vi "calibrationSpectrometer_acceptCommand_Enable.vi"(8 "error in (no error)":errorcluster, 11 "command_Enable_Ctl":T1) -> (0 "error out":errorcluster, 2 "function return":i32, 3 "command_Enable_Ctl out":T1)   [LabVIEW 2016, in "SALLV_calibrationSpectrometer.lvlib"]
doc: "int calibrationSpectrometer_shm_acceptCommand_EnableLV(calibrationSpectrometer_command_EnableLV *command_Enable_Ctl );"
uses:
  SALLV_calibrationSpectrometer.lvlib
  DataTypes/command_Enable.ctl
  SALLV_calibrationSpectrometer.so
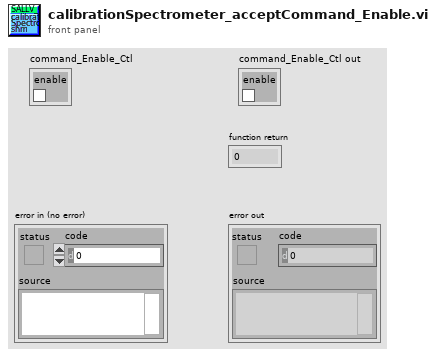
[diagram p1: front panel]
types:
  T1 = typedef "SALLV_calibrationSpectrometer.lvlib/command_Enable.ctl" = cluster{"enable":bool}
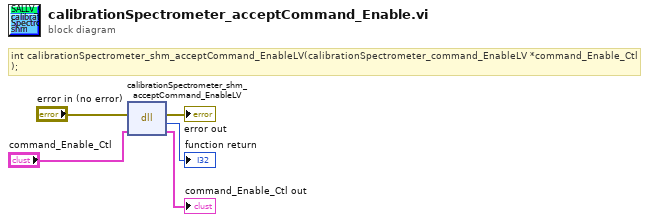
[diagram p0: block diagram]
diagram:
  # "int calibrationSpectrometer_shm_acceptCommand_EnableLV(calibrationSpectrometer_command_EnableLV *command_Enable_Ctl );"
  n1 = dll-call lib="home/harini/TCS/sallv_sedspectrometer/SALLV_calibrationSpectrometer.*" fn="calibrationSpectrometer_shm_acceptCommand_EnableLV"(error in="error in (no error)", "command_Enable_Ctl"="command_Enable_Ctl") -> (error out=→"error out":errorcluster, →"function return":i32, "command_Enable_Ctl"=→"command_Enable_Ctl out":T1)  [unwired: 2 in, 1 out]
